vi "Concatenador_tipo_dadoSuper.vi"(0 "Tipo de Dado(SPW)":T1 items=["Engenharia", "Puro(mA)"], 5 "Tipo de Dado(SPK)":T1 items=["Engenharia", "Puro(mA)"], 7 "Tipo de Dado(SKM)":T1 items=["Engenharia", "Puro(mA)"], 9 "Tipo de Dado(SKI)":T1 items=["Engenharia", "Puro(mA)"], 11 "Tipo de Dado(SKS)":T1 items=["Engenharia", "Puro(mA)"]) -> (8 "Tipo de Dado(Final)":T1 items=["Engenharia", "Puro(mA)"])   [LabVIEW 2019]
uses:
  \\SERVERPC\Server/padrao_tipo_dado.ctl
panel:
  out "TD-anterior":T1 items=["Engenharia", "Puro(mA)"]
  out "anterior":i16
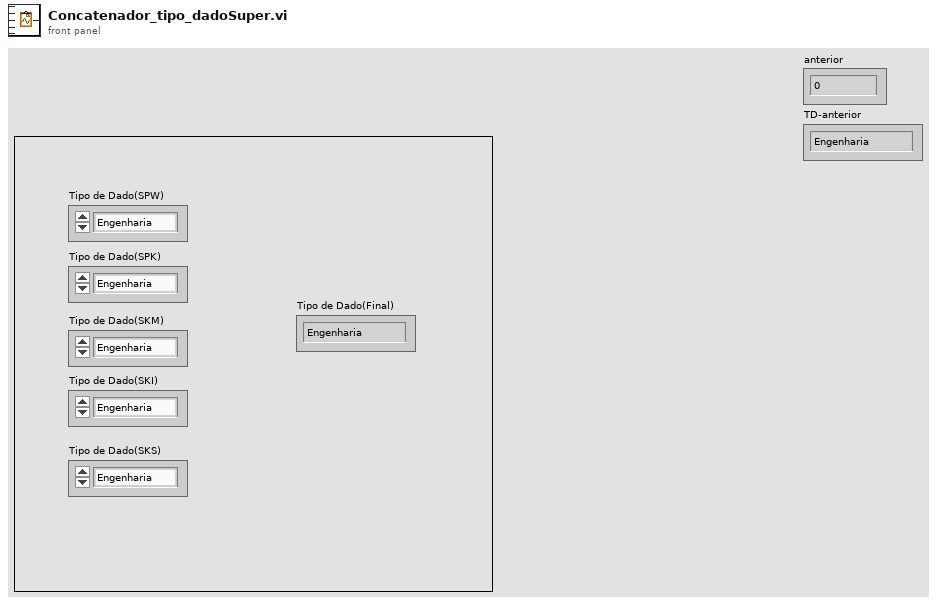
[diagram p1: front panel]
types:
  T1 = typedef "padrao_tipo_dado.ctl" = u16
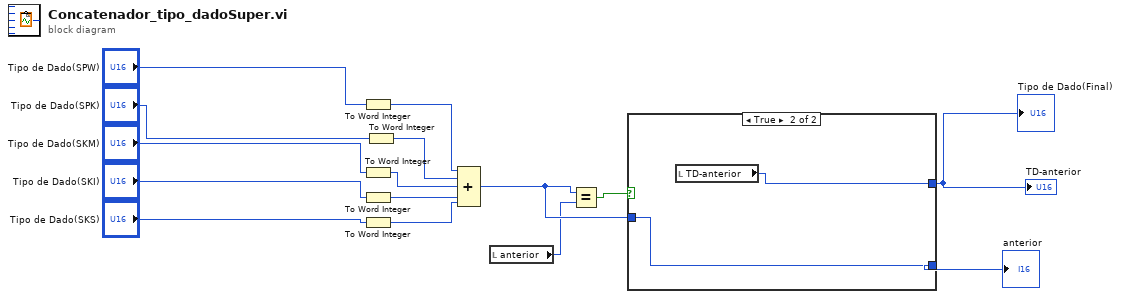
[diagram p0: block diagram]
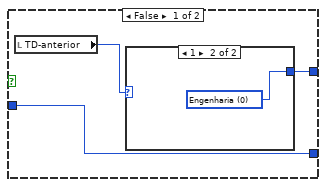
[diagram p2: hidden frame]
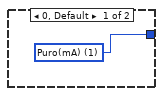
[diagram p3: hidden frame]
diagram:
  n1 = To Word Integer(number="Tipo de Dado(SPW)") -> (16bit integer=w14:i16)
  n2 = To Word Integer(number="Tipo de Dado(SKM)") -> (16bit integer=w8:i16)
  n3 = To Word Integer(number="Tipo de Dado(SKI)") -> (16bit integer=w7:i16)
  n4 = To Word Integer(number="Tipo de Dado(SKS)") -> (16bit integer=w6:i16)
  n5 = To Word Integer(number="Tipo de Dado(SPK)") -> (16bit integer=w9:i16)
  n6 = Compound Arithmetic op=ADD(w14, w9, w8, w7, w6) -> (w4:i16)
  n7 = local read "anterior"() -> (w3:i16)
  n8 = Equal?(x=w4, y=w3) -> (x = y?=w2:bool)
  n9 = case shown="True" w2 {
    tunnel: w4 -> [w18 w22]
    tunnel: [w18 w22] -> w5
    tunnel: [w16 w21] -> w1
    frame False {
      n10 = local read "TD-anterior"() -> (w17:T1)
      n11 = case shown="1" w17 {
        tunnel: [w19 w20] -> w16
        frame 0, Default {
          w19 = T1 1 items=["Engenharia", "Puro(mA)"] ("Tipo de Dado(Final)")
        }
        frame 1 {
          w20 = T1 0 items=["Engenharia", "Puro(mA)"] ("Tipo de Dado(Final)")
        }
      }
    }
    frame True {
      n12 = local read "TD-anterior"() -> (w21:T1)
    }
  }
  "Tipo de Dado(Final)" <- w1
  "anterior" <- w5
  "TD-anterior" <- w1
